vi "dfd_Check FIR Coefficient Length.vi"(7 "#coefficients length":i32, 8 "error in (no error)":errorcluster, 11 "coefficients in":dbl[](array[numeric])) -> (0 "error out":errorcluster, 3 "coefficients out":dbl[](array[numeric]))   [LabVIEW 2017, in "NI_DigFilter_CodeGen.lvlib"]
uses:
  <vilib>/addons/Digital Filter Design/NI_DigFilter_CodeGen.lvlib
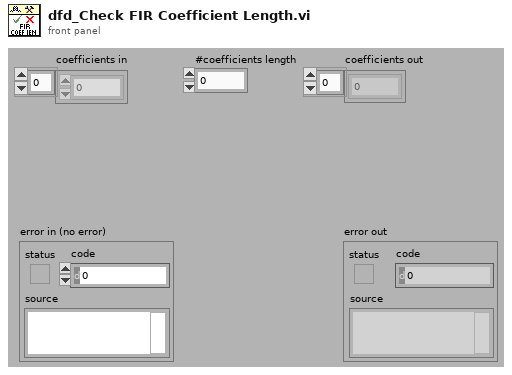
[diagram p1: front panel]
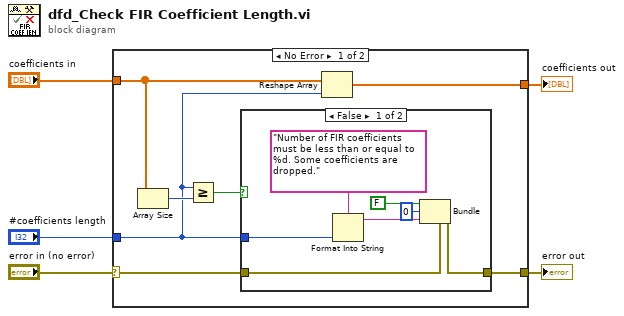
[diagram p0: block diagram]
diagram:
  n1 = case shown="No Error" "error in (no error)" {
    selector: "error in (no error)" -> [w12 w21]
    tunnel: "#coefficients length" -> [w6 _]
    tunnel: "coefficients in" -> [w8 _]
    tunnel: [w7 _] -> w2
    tunnel: [w11 w21] -> w1
    frame No Error {
      n2 = Array Size(array=w8) -> (size(s)=w10:i32)
      n3 = Greater Or Equal?(x=w6, y=w10) -> (x >= y?=w9:bool)
      n4 = case shown="False" w9 {
        tunnel: w12 -> [w19 w20]
        tunnel: [w18 w20] -> w11
        tunnel: w6 -> [w13 _]
        frame False {
          n5 = Format Into String(format string="Number of FIR coefficients must be less than or equal to %d. Some coefficients are dropped.", w13) -> (resulting string=w14:string)  [unwired: 2 in, 1 out]
          n6 = Bundle(cluster=w19, "status"=FALSE, "code"=0, "source"=w14) -> (w18:errorcluster)
        }
        frame True {
        }
      }
      n7 = Reshape Array(w8, w6) -> (w7:dbl[])
    }
    frame Error {
    }
  }
  "error out" <- w1
  "coefficients out" <- w2
